vi "Create Analog Replay.vi"(8 "error in (no error)":errorcluster, 10 "analog replay name":string, 11 "Section Ptr":T1 format="%.0x") -> (0 "error out":errorcluster, 2 "Analog replay ref":T1 format="%.0x", 3 "Section Ptr dup":T1 format="%.0x")   [LabVIEW 2013, in "Engine Simulation Toolkit System Explorer.lvlib"]
uses:
  Engine Simulation Toolkit System Explorer.lvlib
  <vilib>/NI Veristand/Custom Device API/Custom Device Item Ref.ctl
  <vilib>/NI Veristand/Custom Device API/Custom Device Channel Type.ctl
  Shared/Constants and GUIDs.vi
  Shared/Properties.vi
  <vilib>/NI Veristand/Custom Device API/Set Item Property (String).vi
  Shared/Engine Simulation Toolkit Shared.lvlib
  <vilib>/NI Veristand/Custom Device API/Custom Device API.lvlib
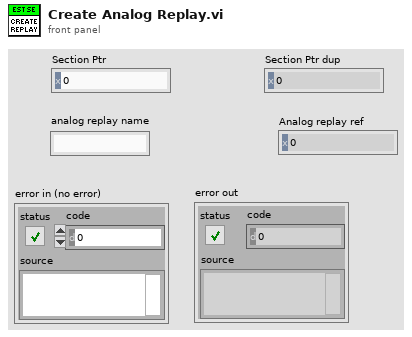
[diagram p1: front panel]
types:
  T1 = typedef "Custom Device API.lvlib/Custom Device Item Ref.ctl" = u64
  T2 = typedef "Custom Device API.lvlib/Custom Device Channel Type.ctl" = enum16{"Input", "Output"}
  T3 = typedef "Engine Simulation Toolkit Shared.lvlib/Channel.ctl" = cluster{"Name":string, "Units":string, "Default":dbl, "Description":string}
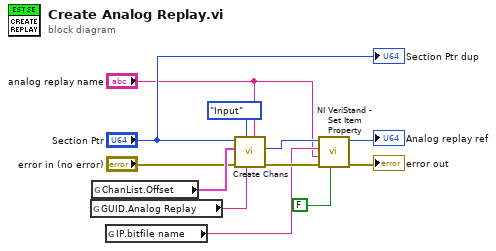
[diagram p0: block diagram]
diagram:
  n1 = global read "Constants and GUIDs.vi" "GUID.Analog Replay"() -> (w10:string)
  n2 = global read "Constants and GUIDs.vi" "ChanList.Offset"() -> (w11:T3[])
  n3 = global read "Properties.vi" "IP.bitfile name"() -> (w4:string)
  n4 = call "Create Chans.vi"("New Section Name (none)"="analog replay name", "new section GUID (\"\":del prot)"=w10, "Type"=Custom_Device_Channel_Type."Input", "error in (no error)"="error in (no error)", "Channels"=w11, "Section Ptr"="Section Ptr") -> ("error out"=w9:errorcluster, "new section ref"=w5:T1)  [unwired: 2 in, 2 out]
  n5 = call-poly <vilib>:"NI VeriStand - Set Item Property.vi"("Binary String (T)"=FALSE, "error in (no error)"=w9, "Value"="analog replay name", "Property Name"=w4, "Item Ref in"=w5) -> ("error out"=→"error out":errorcluster, "Item Ref out"=→"Analog replay ref":T1)  [unwired: 4 in, 1 out]
  "Section Ptr dup" <- "Section Ptr"
